vi "CRYDV Get LIST.vi"(0 "sAction":string="asada", 1 "DataView Array Index":i32, 2 "List_In":cluster{"nID":i32, "pVIRef":refnum<vi>}[](array[cluster]), 3 "MousePos":T1, 4 "SubPanel array":refnum<vi>[](array[refnum])) -> (7 "List_Out":cluster{"nID":i32, "pVIRef":refnum<vi>}[](array[cluster]), 8 "pVIRef_Out":refnum<vi>, 9 "nData_Out":i32, 10 "bResult":bool=TRUE)   [LabVIEW 2013]
uses:
  CRYNew View Global.vi
panel:
  out "Max":i32
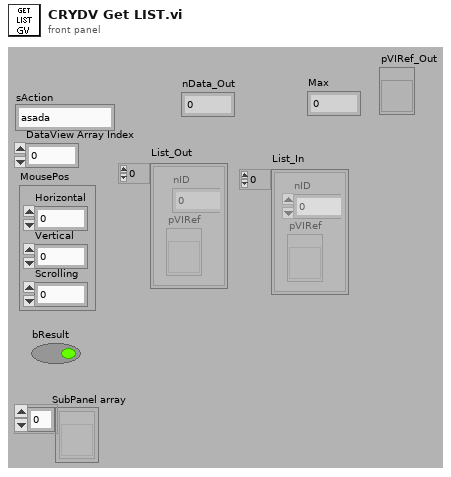
[diagram p1: front panel]
types:
  T1 = cluster{"Horizontal":i32, "Vertical":i32, "Scrolling":i32}
  T2 = typedef "Graph Main Info Cluster.ctl" = cluster{"Selected_BarIdx":i32, "Selected_PanelIdx":i32, "Graph Main VIRef":refnum<vi>, "ToolBarClick":bool, "Spliter Ref Array":refnum<vi>[], "Panel Ref Array":refnum<vi>[], "Spliter_matrix":i32[][], "Panel_matrix":i32[][], "child_spliterIdx_matrix":i32[][], "split_pos_matrix":i32[][], "Title State":bool, "sQueueName":string, "Frame nID":i32, "Graph VIRef Array":cluster{"Graph VIRef":refnum<vi>, "Panel Idx":i32, "Frame VIRef":refnum<vi>, "Icon Ring":i32, "Graph Type":string}[], "View Type":string}
  T3 = enum32{"Invalid", "Standard", "Closed", "Hidden", "Minimized", "Maximized"}
  T4 = typedef "LVRectTypeDef.ctl" = cluster{"Left":i16, "Top":i16, "Right":i16, "Bottom":i16}
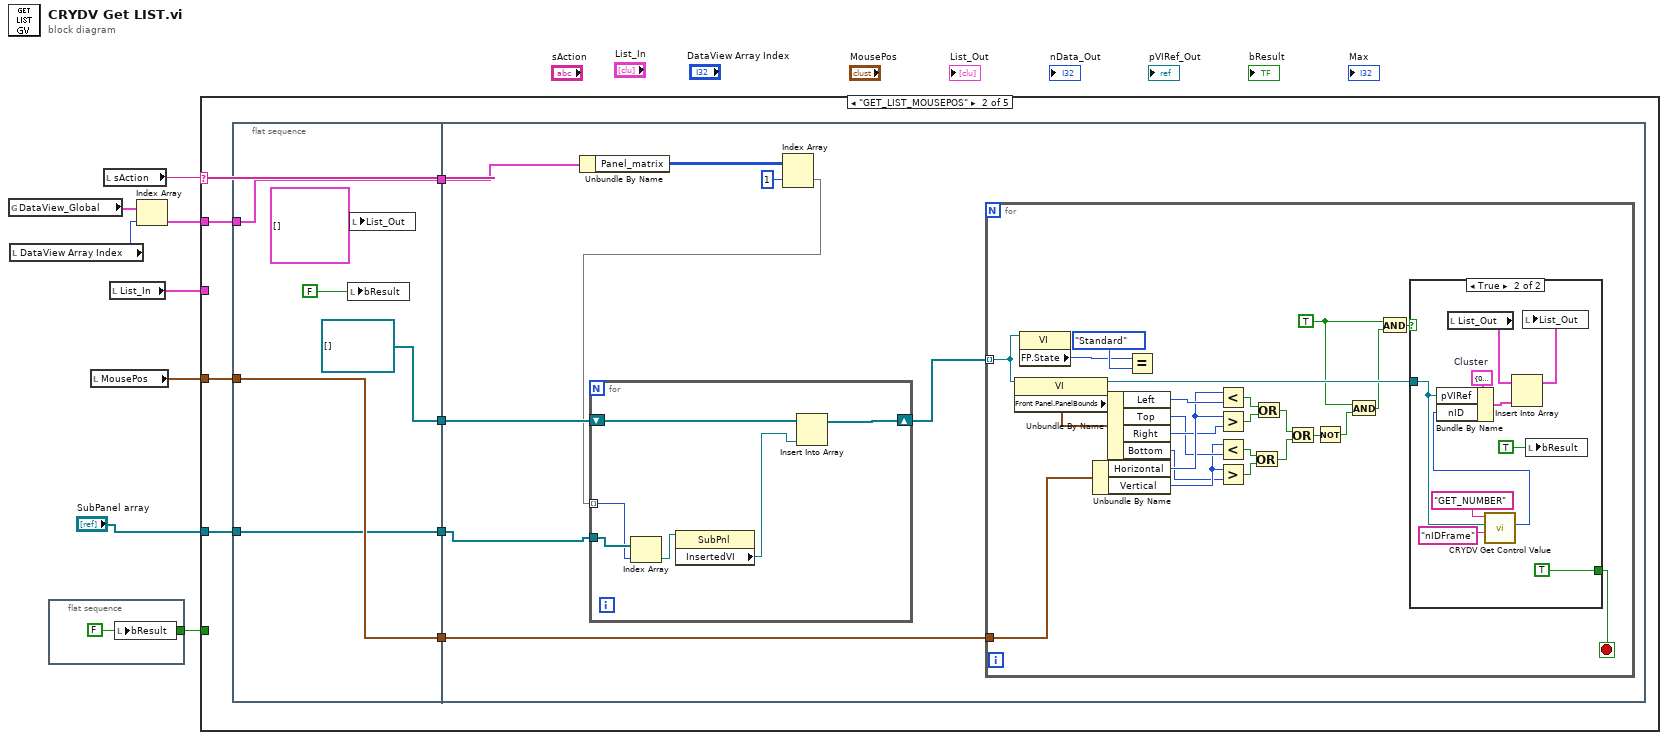
[diagram p0: block diagram]
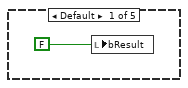
[diagram p2: hidden frame]
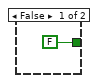
[diagram p3: hidden frame]
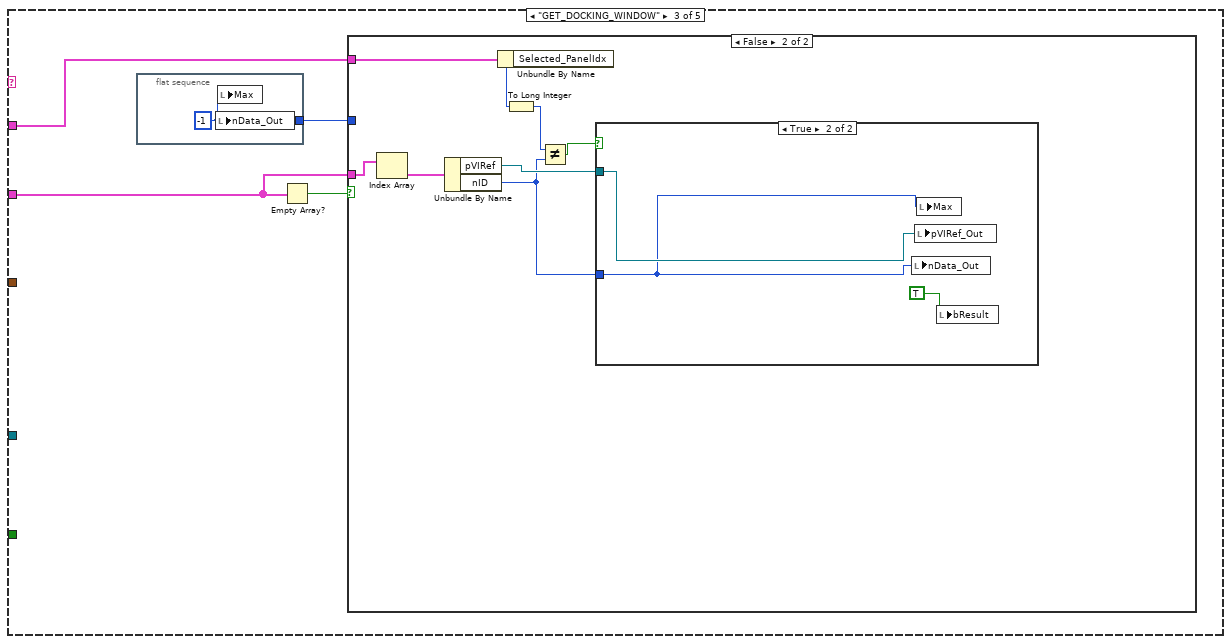
[diagram p4: hidden frame]
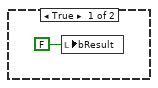
[diagram p5: hidden frame]
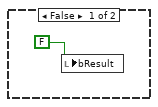
[diagram p6: hidden frame]
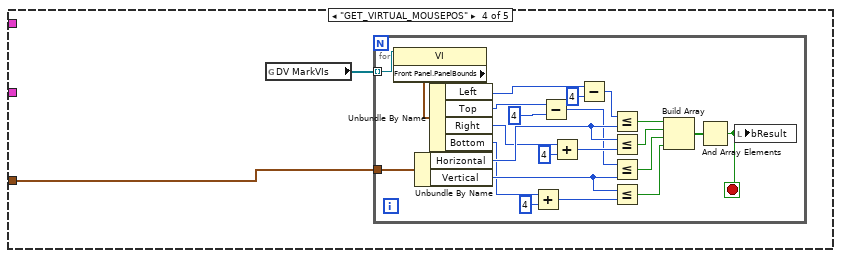
[diagram p7: hidden frame]
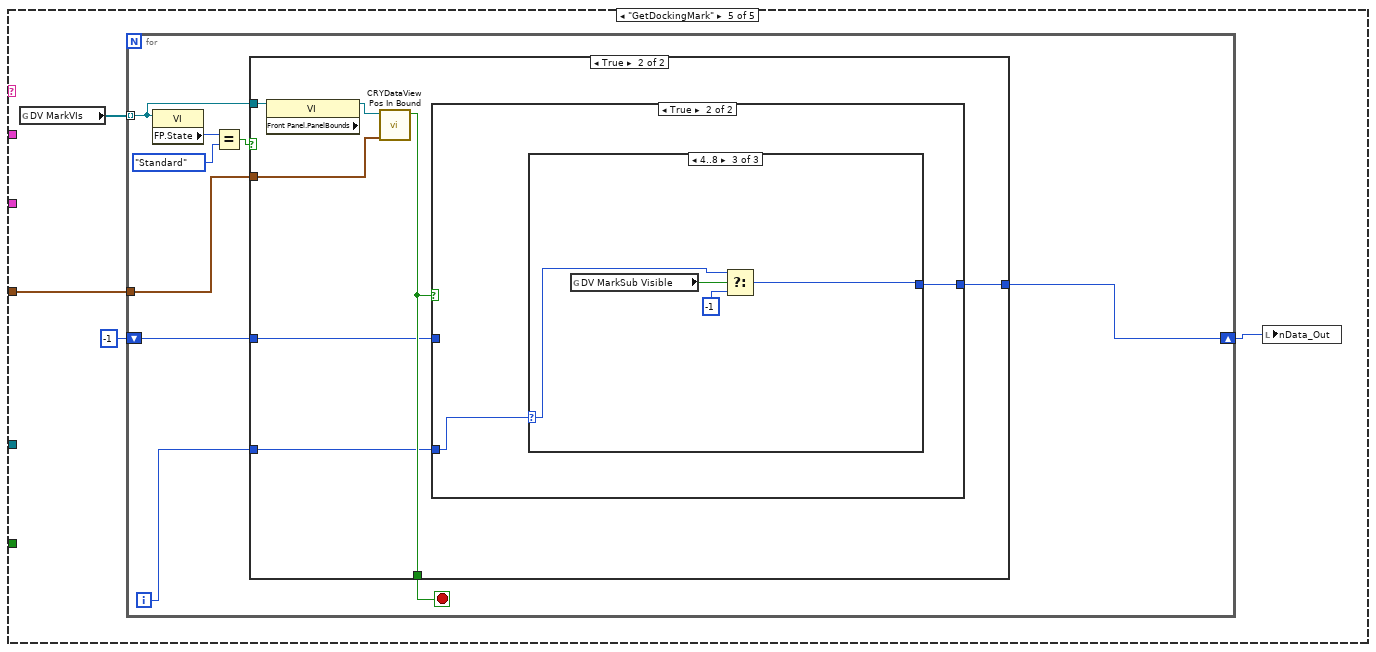
[diagram p8: hidden frame]
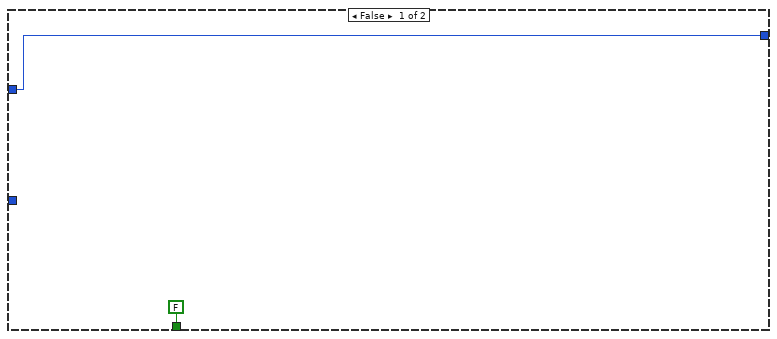
[diagram p9: hidden frame]
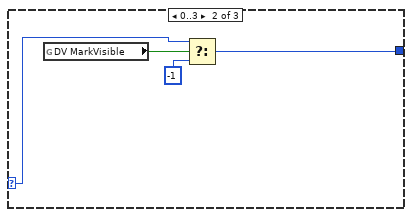
[diagram p12: hidden frame]
diagram:
  n1 = global read "CRYNew View Global.vi" "DataView_Global"() -> (w1:T2[])
  n2 = local read "DataView Array Index"() -> (w5:i32)
  n3 = flat-sequence {
    tunnel: [w9] -> w3
    frame #0 {
      w9 = FALSE ("bResult")
      n4 = local write "bResult"(w9) -> ()
    }
  }
  n5 = local read "MousePos"() -> (w7:T1)
  n6 = local read "sAction"() -> (w8:string)
  n7 = local read "List_In"() -> (w6:cluster{"nID":i32, "pVIRef":refnum<vi>}[])
  n8 = Index Array(array=w1, index=w5) -> (element=w4:T2)
  n9 = case shown="\"GET_LIST_MOUSEPOS\"" w8 {
    tunnel: w7 -> [_ w17 _ w91 w118]
    tunnel: w6 -> [_ _ w76 _ _]
    tunnel: w4 -> [_ w13 w74 _ _]
    tunnel: w3 -> [_ _ _ _ _]
    tunnel: "SubPanel array" -> [_ w11 _ _ _]
    frame Default {
      n10 = local write "bResult"(FALSE ("bResult")) -> ()
    }
    frame "GET_LIST_MOUSEPOS" {
      n11 = flat-sequence {
        tunnel: w17 -> [w23]
        tunnel: [w23] -> w16
        tunnel: [refnum<vi>[] [] ("List_Out")] -> w15
        tunnel: [w19] -> w14
        tunnel: w13 -> [w19]
        tunnel: [w18] -> w12
        tunnel: w11 -> [w18]
        tunnel: w16 -> [w31]
        tunnel: w15 -> [w30]
        tunnel: w14 -> [w28]
        tunnel: w12 -> [w25]
        frame #0 {
          n12 = local write "bResult"(FALSE ("bResult")) -> ()
          n13 = local write "List_Out"(cluster{"nID":i32, "pVIRef":refnum<vi>}[] [] ("List_Out")) -> ()
        }
        frame #1 {
          n14 = Unbundle By Name(w28) -> ("Panel_matrix"=w24:i32[][])
          n15 = Index Array(array=w24, index (row)=1) -> (element=w26:i32[])  [unwired: 1 in]
          n16 = for {
            tunnel: w26 -> [w34] mode=indexing
            shift-right: [w36] -> w29
            shift-left: w30 -> [w37]
            tunnel: w25 -> [w35]
            n17 = Index Array(array=w35, index=w34) -> (element=w33:refnum<vi>)
            n18 = property class="SubPnl"(reference=w33) -> ("InsertedVI"=w32:refnum<vi>)  [unwired: 1 in, 2 out]
            n19 = Insert Into Array(array=w37, new element=w32) -> (w36:refnum<vi>[])  [unwired: 1 in]
          }
          n20 = for {
            tunnel: w31 -> [w61]
            tunnel: w29 -> [w40] mode=indexing
            stop <- w38 stop-if-true
            w39 = TRUE
            n21 = property class="VI"(reference=w40) -> (reference out=w57:refnum<vi>, "Front Panel.PanelBounds"=w60:T4)  [unwired: 1 in, 1 out]
            n22 = property class="VI"(reference=w40) -> ("FP.State"=w58:T3)  [unwired: 1 in, 2 out]
            n23 = Unbundle By Name(w61) -> ("Horizontal"=w55:i32, "Vertical"=w52:i32)
            n24 = Unbundle By Name(w60) -> ("Left"=w56:i16, "Top"=w53:i16, "Right"=w54:i16, "Bottom"=w51:i16)
            n25 = Equal?(x=w58, y=T3."Standard" ("Front Panel Window:State")) -> ()  [unwired: 1 out]
            n26 = Less?(x=w55, y=w56) -> (x < y?=w49:bool)
            n27 = Greater?(x=w55, y=w54) -> (0:w50:bool)
            n28 = Less?(x=w52, y=w53) -> (x < y?=w48:bool)
            n29 = Greater?(x=w52, y=w51) -> (0:w47:bool)
            n30 = Or(x=w48, y=w47) -> (x .or. y?=w45:bool)
            n31 = Or(x=w49, y=w50) -> (x .or. y?=w46:bool)
            n32 = Or(x=w46, y=w45) -> (x .or. y?=w44:bool)
            n33 = Not(x=w44) -> (.not. x?=w43:bool)
            n34 = And(x=w39, y=w43) -> (x .and. y?=w41:bool)
            n35 = And(x=w39, y=w41) -> (x .and. y?=w42:bool)
            n36 = case shown="True" w42 {
              tunnel: w57 -> [_ w65]
              tunnel: [FALSE TRUE] -> w38
              frame False {
              }
              frame True {
                w69 = cluster{"nID":i32, "pVIRef":refnum<vi>} {"nID"=0, "pVIRef"=refnum}  # Cluster
                n37 = local read "List_Out"() -> (w72:cluster{"nID":i32, "pVIRef":refnum<vi>}[])
                n38 = call "CRYDV Get Control Value.vi"("sControlName"="nIDFrame", "pVIRef"=w65, "sAction"="GET_NUMBER") -> ("Numeric"=w64:i32)  [unwired: 4 in, 4 out]
                n39 = Bundle By Name(cluster=w69, "pVIRef"=w65, "nID"=w64) -> (w68:cluster{"nID":i32, "pVIRef":refnum<vi>})
                n40 = Insert Into Array(array=w72, new element=w68) -> (w71:cluster{"nID":i32, "pVIRef":refnum<vi>}[])  [unwired: 1 in]
                n41 = local write "List_Out"(w71) -> ()
                n42 = local write "bResult"(TRUE ("bResult")) -> ()
              }
            }
          }
        }
      }
    }
    frame "GET_DOCKING_WINDOW" {
      n43 = flat-sequence {
        tunnel: [w77] -> w73
        frame #0 {
          w77 = -1 ("nData")
          n44 = local write "nData_Out"(w77) -> ()
          n45 = local write "Max"(w77) -> ()
        }
      }
      n46 = Empty Array?(array=w76) -> (empty?=w75:bool)
      n47 = case shown="False" w75 {
        tunnel: w76 -> [_ w81]
        tunnel: w74 -> [_ w86]
        tunnel: w73 -> [_ _]
        frame True {
          n48 = local write "bResult"(FALSE ("bResult")) -> ()
        }
        frame False {
          n49 = Index Array(array=w81) -> (element=w82:cluster{"nID":i32, "pVIRef":refnum<vi>})  [unwired: 1 in]
          n50 = Unbundle By Name(w82) -> ("pVIRef"=w84:refnum<vi>, "nID"=w83:i32)
          n51 = Unbundle By Name(w86) -> ("Selected_PanelIdx"=w80:i32)
          n52 = To Long Integer(number=w80) -> (32bit integer=w79:i32)
          n53 = Not Equal?(x=w79, y=w83) -> (x != y?=w85:bool)
          n54 = case shown="True" w85 {
            tunnel: w84 -> [_ w90]
            tunnel: w83 -> [_ w88]
            frame False {
              n55 = local write "bResult"(FALSE ("bResult")) -> ()
            }
            frame True {
              n56 = local write "nData_Out"(w88) -> ()
              n57 = local write "pVIRef_Out"(w90) -> ()
              n58 = local write "Max"(w88) -> ()
              n59 = local write "bResult"(TRUE ("bResult")) -> ()
            }
          }
        }
      }
    }
    frame "GET_VIRTUAL_MOUSEPOS" {
      n60 = global read "CRYNew View Global.vi" "DV MarkVIs"() -> (w92:refnum<vi>[])
      n61 = for {
        tunnel: w91 -> [w96]
        tunnel: w92 -> [w95] mode=indexing
        stop <- w94 stop-if-true
        n62 = property class="VI"(reference=w95) -> ("Front Panel.PanelBounds"=w113:T4)  [unwired: 1 in, 2 out]
        n63 = Unbundle By Name(w96) -> ("Horizontal"=w115:i32, "Vertical"=w114:i32)
        n64 = Unbundle By Name(w113) -> ("Left"=w100:i16, "Top"=w98:i16, "Right"=w102:i16, "Bottom"=w104:i16)
        n65 = Add(x=w104, y=4) -> (x+y=w103:i32)
        n66 = Subtract(x=w98, y=4) -> (x-y=w97:i32)
        n67 = Add(x=w102, y=4) -> (x+y=w101:i32)
        n68 = Subtract(x=w100, y=4) -> (x-y=w99:i32)
        n69 = Less Or Equal?(x=w99, y=w115) -> (x <= y?=w112:bool)
        n70 = Less Or Equal?(x=w115, y=w101) -> (x <= y?=w111:bool)
        n71 = Less Or Equal?(x=w97, y=w114) -> (x <= y?=w110:bool)
        n72 = Less Or Equal?(x=w114, y=w103) -> (x <= y?=w109:bool)
        n73 = Build Array(w112, w111, w110, w109) -> (w108:bool[])
        n74 = And Array Elements(Boolean array=w108) -> (logical AND=w94:bool)
        n75 = local write "bResult"(w94) -> ()
      }
    }
    frame "GetDockingMark" {
      n76 = global read "CRYNew View Global.vi" "DV MarkVIs"() -> (w119:refnum<vi>[])
      n77 = for {
        tunnel: w119 -> [w125] mode=indexing
        tunnel: w118 -> [w124]
        shift-right: [w121] -> w116
        shift-left: -1 -> [w120]
        i -> [w122]
        stop <- w123 stop-if-true
        n78 = property class="VI"(reference=w125) -> ("FP.State"=w128:T3)  [unwired: 1 in, 2 out]
        n79 = Equal?(x=w128, y=T3."Standard" ("Front Panel Window:State")) -> (x = y?=w126:bool)
        n80 = case shown="True" w126 {
          tunnel: w125 -> [_ w137]
          tunnel: w124 -> [_ w135]
          tunnel: [FALSE ("bResult") w134] -> w123
          tunnel: w122 -> [_ w133]
          tunnel: [w129 w132] -> w121
          tunnel: w120 -> [w129 w131]
          frame False {
          }
          frame True {
            n81 = property class="VI" props=["Front Panel.PanelBounds"](reference=w137) -> (reference out=w136:refnum<vi>)  [unwired: 1 in, 2 out]
            n82 = call "CRYDataView Pos In Bound.vi"("Mouse Pos"=w135, "Ref In"=w136) -> ("bResult"=w134:bool)  [unwired: 9 in]
            n83 = case shown="True" w134 {
              tunnel: w133 -> [_ w140]
              tunnel: [w138 w139] -> w132
              tunnel: w131 -> [w138 _]
              frame False {
              }
              frame True {
                n84 = case shown="4..8" w140 {
                  selector: w140 -> [w141 w143 w146]
                  tunnel: [w141 w142 w147] -> w139
                  frame Default {
                  }
                  frame 0..3 {
                    n85 = global read "CRYNew View Global.vi" "DV MarkVisible"() -> (w145:bool)
                    n86 = Select(t=w143, s=w145, f=-1) -> (s? t:f=w142:i32)
                  }
                  frame 4..8 {
                    n87 = global read "CRYNew View Global.vi" "DV MarkSub Visible"() -> (w149:bool)
                    n88 = Select(t=w146, s=w149, f=-1) -> (s? t:f=w147:i32)
                  }
                }
              }
            }
          }
        }
      }
      n89 = local write "nData_Out"(w116) -> ()
    }
  }
